vi "SendData.vi"(8 "error in (no error)":errorcluster, 9 "timeout ms (100)":i32=100, 10 "data":cdb[](array[numeric]), 11 "reference in":refnum<class "NS slave.lvclass">) -> (0 "error out":errorcluster, 1 "timed out?":bool, 3 "reference out":refnum<class "NS slave.lvclass">)   [LabVIEW 2019, in "CommandResponse communication.lvlib" / "NS slave.lvclass"]
doc: "Write data stream to network stream"
uses:
  NS slave.lvclass
  C:/Barkhausen mmWave radar/Development/LV/Barkhausen mmWave hardware control/Host/Intertarget communication/CR slave_class/CR slave.lvclass
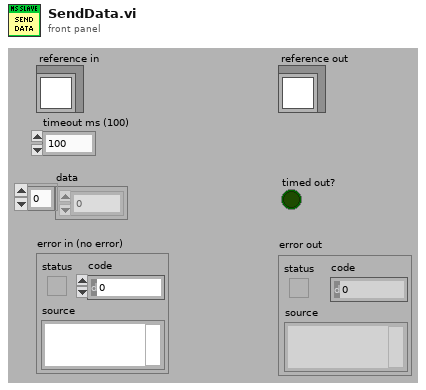
[diagram p1: front panel]
types:
  T1 = typedef "CommandResponse communication.lvlib/NS slave.lvclass/ObjectAttributes.ctl" = cluster{"connected":bool, "stop":bool, "ID":string, "command rd":refnum<k21>, "response wr":refnum<k21>, "data wr":refnum<k21>}
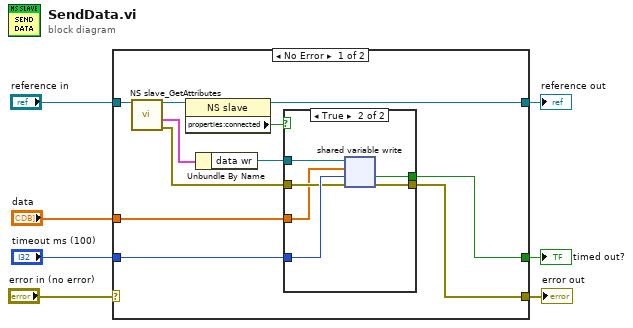
[diagram p0: block diagram]
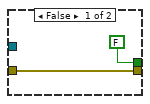
[diagram p2: hidden frame]
diagram:
  n1 = case shown="No Error" "error in (no error)" {
    selector: "error in (no error)" -> [_ w28]
    tunnel: [w11 w28] -> w6
    tunnel: [w9 w27] -> w4
    tunnel: "reference in" -> [w16 w27]
    tunnel: "timeout ms (100)" -> [w14 _]
    tunnel: [w13 _] -> w2
    tunnel: "data" -> [w10 _]
    frame No Error {
      n2 = call "NS slave_GetAttributes.vi"("reference in"=w16) -> ("error out"=w12:errorcluster, "attributes"=w17:T1, "reference out"=w18:refnum<class "NS slave.lvclass">)  [unwired: 7 in, 1 out]
      n3 = property class="NS slave"(reference=w18) -> (reference out=w9:refnum<class "NS slave.lvclass">, "properties:connected"=w8:bool)  [unwired: 1 in, 1 out]
      n4 = Unbundle By Name(w17) -> ("data wr"=w15:refnum<k21>)
      n5 = case shown="True" w8 {
        tunnel: w15 -> [_ w26]
        tunnel: w14 -> [_ w25]
        tunnel: [FALSE w24] -> w13
        tunnel: w12 -> [w20 w23]
        tunnel: [w20 w22] -> w11
        tunnel: w10 -> [_ w21]
        frame False {
        }
        frame True {
          n6 = shared-variable-write(w26, w23, w21, w25) -> (w22:errorcluster, w24:bool)  [unwired: 1 out]
        }
      }
    }
    frame Error {
    }
  }
  "error out" <- w6
  "reference out" <- w4
  "timed out?" <- w2
